vi "Read COM.lvclass.vi"(8 "error in (no error)":errorcluster, 11 "Electrometer in":refnum<class "Electrometer.lvclass">) -> (0 "error out":errorcluster, 2 "VISA":refnum<visa-resource-name>, 3 "Electrometer out":refnum<class "Electrometer.lvclass">)   [LabVIEW 2016, in "Electrometer.lvclass"]
uses:
  Electrometer.lvclass
  Electrometer.lvclass/Electrometer.ctl
  ElectrometerConfiguration.lvclass
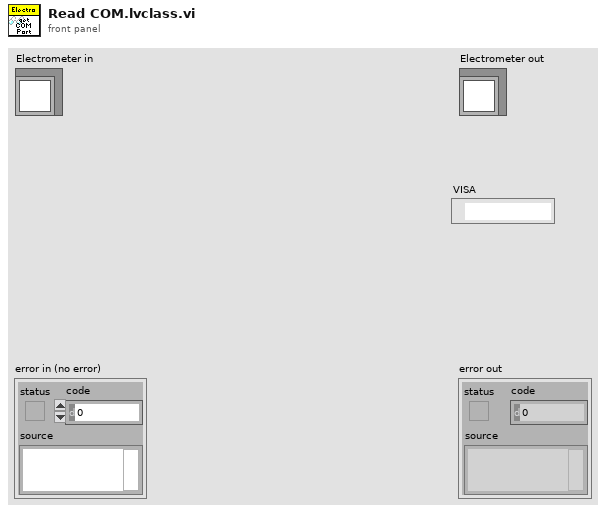
[diagram p1: front panel]
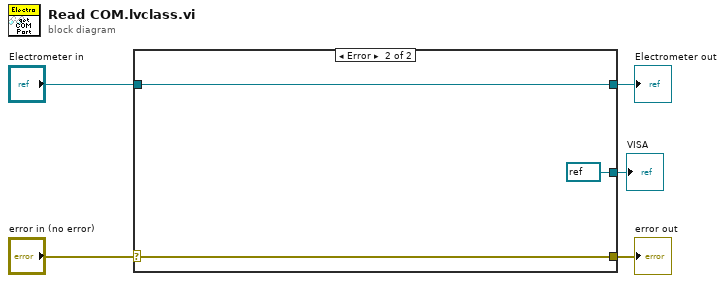
[diagram p0: block diagram]
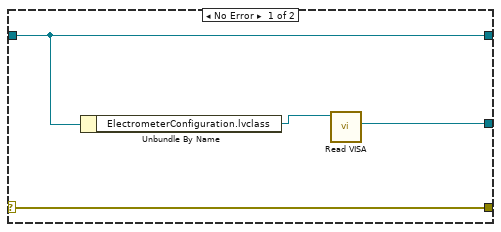
[diagram p2: hidden frame]
diagram:
  n1 = case shown="Error" "error in (no error)" {
    selector: "error in (no error)" -> [w9 w11]
    tunnel: [w9 w11] -> w4
    tunnel: [w8 w12] -> w2
    tunnel: "Electrometer in" -> [w8 w12]
    tunnel: [w6 refnum<visa-resource-name> refnum ("VISA")] -> w1
    frame No Error {
      n2 = Unbundle By Name(w8) -> ("ElectrometerConfiguration.lvclass"=w7:refnum<class "ElectrometerConfiguration.lvclass">)
      n3 = call-dynamic "Read VISA.vi"("ElectrometerConfiguration in"=w7) -> ("VISA"=w6:refnum<visa-resource-name>)  [unwired: 8 in, 2 out]
    }
    frame Error {
    }
  }
  "error out" <- w4
  "Electrometer out" <- w2
  "VISA" <- w1
